vi "Board_Type_Strings.vi"(0 "Board type":T1) -> (1 "Board String":string, 2 "Acquisition VI Name":string)   [LabVIEW 2010]
uses:
  Board_Types.ctl
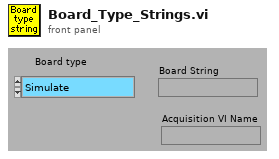
[diagram p1: front panel]
types:
  T1 = typedef "Board_Types.ctl" = enum16{"Simulate", "NB-MIO-16H", "PCI-MIO-16E", "6000E Series", "USB-92xx", "ADC488", "Lab-NB", "NB-DIO-24", "NI-DAQmx", "Local ADAM", "Server Channels"}
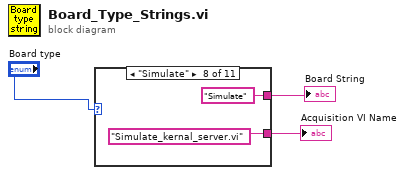
[diagram p0: block diagram]
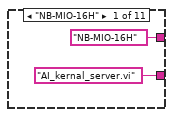
[diagram p2: hidden frame]
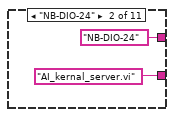
[diagram p3: hidden frame]
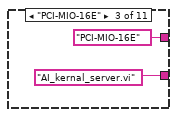
[diagram p4: hidden frame]
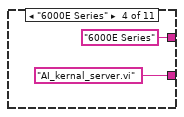
[diagram p5: hidden frame]
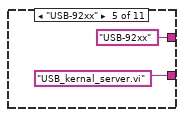
[diagram p6: hidden frame]
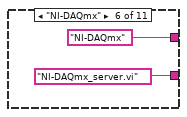
[diagram p7: hidden frame]
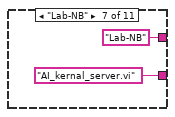
[diagram p8: hidden frame]
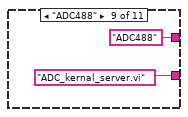
[diagram p9: hidden frame]
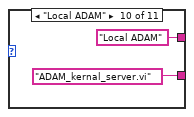
[diagram p10: hidden frame]
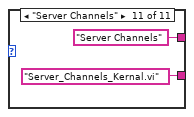
[diagram p11: hidden frame]
diagram:
  n1 = case shown="\"Simulate\"" "Board type" {
    tunnel: ["NB-MIO-16H" "NB-DIO-24" "PCI-MIO-16E" "6000E Series" "USB-92xx" "NI-DAQmx" "Lab-NB" "Simulate" "ADC488" "Local ADAM" "Server Channels"] -> w2
    tunnel: ["AI_kernal_server.vi" "AI_kernal_server.vi" "AI_kernal_server.vi" "AI_kernal_server.vi" "USB_kernal_server.vi" "NI-DAQmx_server.vi" "AI_kernal_server.vi" "Simulate_kernal_server.vi" "ADC_kernal_server.vi" "ADAM_kernal_server.vi" "Server_Channels_Kernal.vi"] -> w1
    frame "NB-MIO-16H" {
    }
    frame "NB-DIO-24" {
    }
    frame "PCI-MIO-16E" {
    }
    frame "6000E Series" {
    }
    frame "USB-92xx" {
    }
    frame "NI-DAQmx" {
    }
    frame "Lab-NB" {
    }
    frame "Simulate" {
    }
    frame "ADC488" {
    }
    frame "Local ADAM" {
    }
    frame "Server Channels" {
    }
  }
  "Board String" <- w2
  "Acquisition VI Name" <- w1
